vi "Bool Name Updater.vi"(8 "error in (no error)":errorcluster, 11 "Cluster In":T1) -> (0 "error out":errorcluster)   [LabVIEW 2018]
uses:
  Shared Controls/Range Updater.ctl
  Val Change Checker.vi
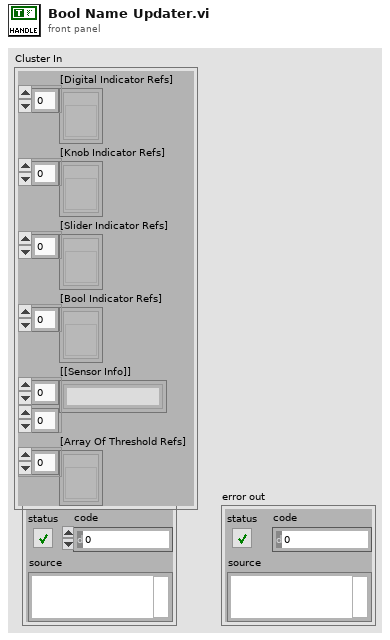
[diagram p1: front panel]
types:
  T1 = typedef "Range Updater.ctl" = cluster{"[Digital Indicator Refs]":refnum<vi>[], "[Knob Indicator Refs]":refnum<vi>[], "[Slider Indicator Refs]":refnum<vi>[], "[Bool Indicator Refs]":refnum<vi>[], "[[Sensor Info]]":string[][], "[Array Of Threshold Refs]":refnum<vi>[]}
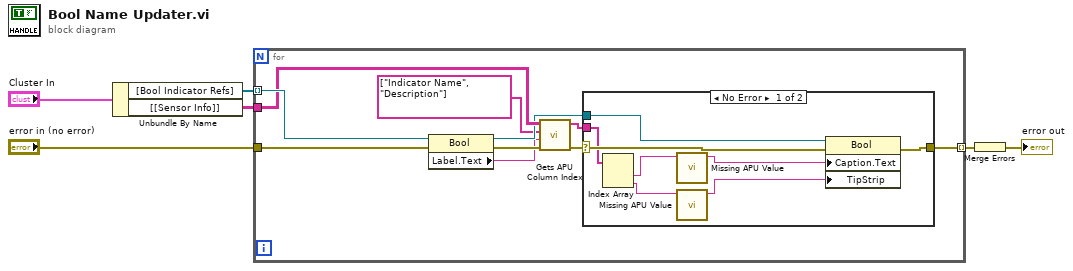
[diagram p0: block diagram]
diagram:
  n1 = Unbundle By Name("Cluster In") -> ("[Bool Indicator Refs]"=w2:refnum<vi>[], "[[Sensor Info]]"=w3:string[][])
  n2 = for {
    tunnel: w2 -> [w16] mode=indexing
    tunnel: w3 -> [w13]
    tunnel: [w14] -> w6 mode=indexing
    tunnel: "error in (no error)" -> [w11]
    n3 = property class="Bool"(reference=w16, error in=w11) -> (reference out=w12:refnum<vi>, error out=w15:errorcluster, "Label.Text"=w7:string)
    n4 = call "Gets APU Column Index.vi"("error in (no error)"=w15, "Tag"=w7, "[Column Names]"=string[] ["Indicator Name", "Description"], "[[Array of Info]]"=w13) -> ("error out"=w10:errorcluster, "[Values out]"=w9:string[])  [unwired: 3 in, 3 out]
    n5 = case shown="No Error" w10 {
      selector: w10 -> [w24 w25]
      tunnel: [w23 w25] -> w14
      tunnel: w12 -> [w22 _]
      tunnel: w9 -> [w21 _]
      frame No Error {
        n6 = Index Array(array=w21) -> (element #1=w20:string, element #2=w18:string)  [unwired: 2 in]
        n7 = call "Missing APU Value.vi"("String In"=w20) -> ("String Out"=w19:string)  [unwired: 8 in, 2 out]
        n8 = call "Missing APU Value.vi"("String In"=w18) -> ("String Out"=w17:string)  [unwired: 8 in, 2 out]
        n9 = property class="Bool"(reference=w22, error in=w24, "Caption.Text"=w19, "TipStrip"=w17) -> (error out=w23:errorcluster)  [unwired: 1 out]
      }
      frame Error {
      }
    }
  }
  n10 = Merge Errors(w6) -> (→"error out":errorcluster)
